vi "2_Temperature_while(170382,170307).vi"() -> ()   [LabVIEW 2015]
panel:
  out "Temperature Graph":dbl[](graph)
  in  "Number of data points":i32
  out "Temperature Chart":dbl(graph)
  in  "Temperature channels":tag="Dev1/ai0"
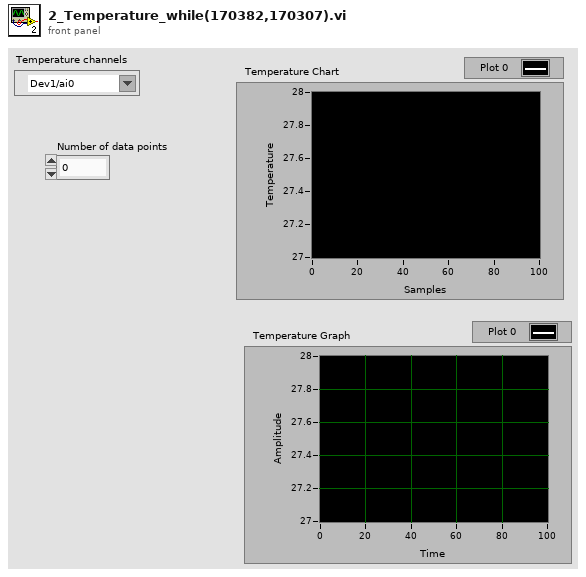
[diagram p1: front panel]
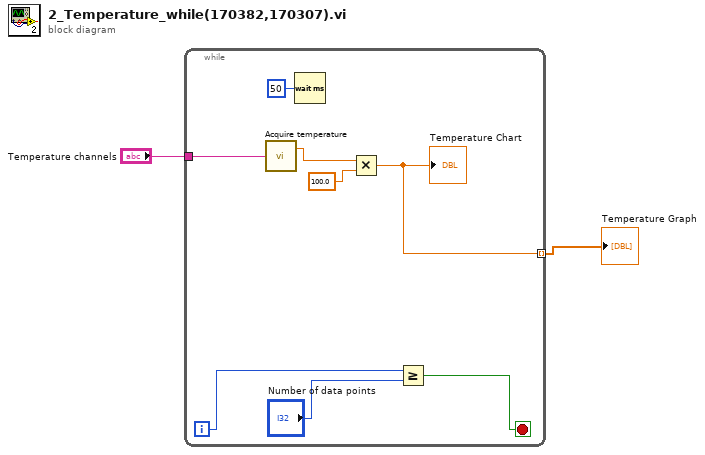
[diagram p0: block diagram]
diagram:
  n1 = while {
    tunnel: "Temperature channels" -> [w10]
    tunnel: [w3] -> w1 mode=indexing
    i -> [w9]
    stop <- w8 stop-if-true
    n2 = call "Acquire temperature.vi"("physical channels"=w10) -> ("data"=w5:dbl)  [unwired: 1 out]
    n3 = Wait (ms)(milliseconds to wait=u32 50) -> ()  [unwired: 1 out]
    n4 = Multiply(x=w5, y=100.0) -> (x*y=w3:dbl)
    "Temperature Chart" <- w3
    n5 = Greater Or Equal?(x=w9, y="Number of data points") -> (x >= y?=w8:bool)
  }
  "Temperature Graph" <- w1
